vi "Supported Smart Syntax Representation.vi"(0 "Message Popup in":refnum<class "Statement.lvclass">, 11 "error in (no error)":errorcluster) -> (4 "Message Popup out":refnum<class "Statement.lvclass">, 6 "Smart Syntax Representation List":string[](array[string]), 15 "error out":errorcluster)   [LabVIEW 2016, in "Statement.lvclass"]
uses:
  Statement.lvclass
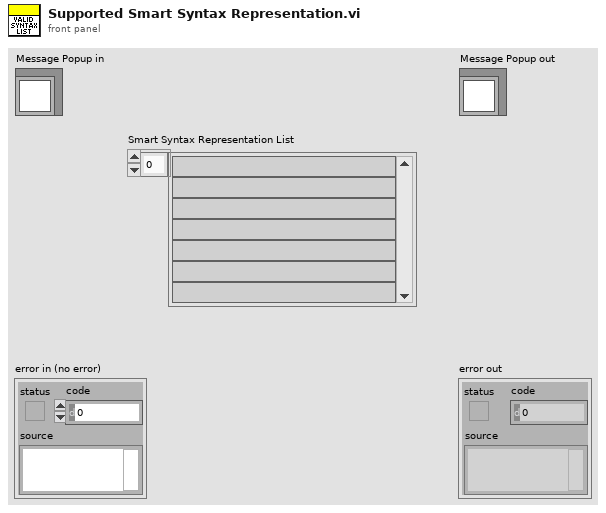
[diagram p1: front panel]
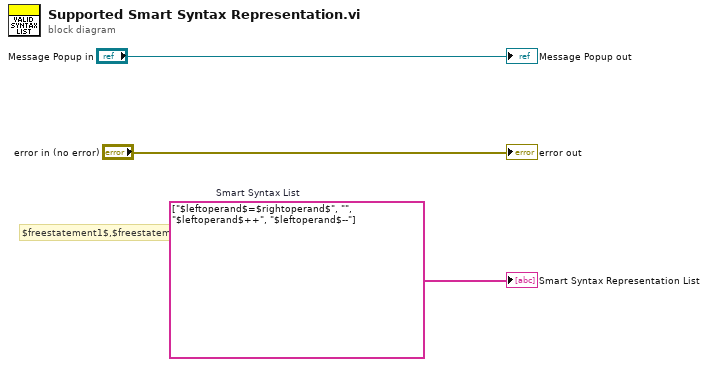
[diagram p0: block diagram]
diagram:
  w1 = string[] ["$leftoperand$=$rightoperand$", "", "$leftoperand$++", "$leftoperand$--"]  # Smart Syntax List
  # "$freestatement1$,$freestatement2$"
  "error out" <- "error in (no error)"
  "Message Popup out" <- "Message Popup in"
  "Smart Syntax Representation List" <- w1
